vi "3Dconfig.vi"(0 "SceneObject in":refnum<vi>, 1 "Proximity Tap":bool, 2 "Weapon":T1(ring), 3 "error in (no error)":errorcluster) -> (5 "SceneObject out":refnum<vi>, 6 "error out":errorcluster)   [LabVIEW 2014]
doc: "Changes the appearance of the lightsaber. Specifically, this VI enables/disables the existing Lightsaber blade and changes the color"
uses:
  <vilib>/picture/3D Picture Control/NI_3D Picture Control.lvlib
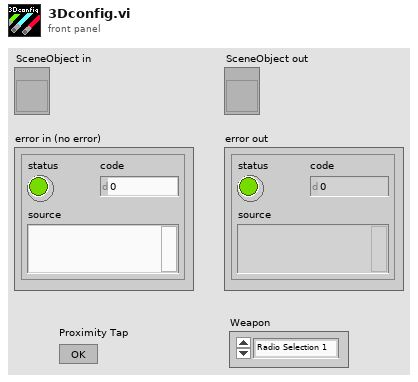
[diagram p1: front panel]
types:
  T1 = enum32{"Radio Selection 1", "Radio Selection 2", "Radio Selection 3", "Radio Selection 4"}
  T2 = enum16{"As a Decal", "With Modulation", "With Blending", "As a replacement"}
  T3 = typedef "imagedata.ctl" = cluster{"image type":i32, "image depth":i32, "image":u8[], "mask":u8[], "colors":u32[], "Rectangle":cluster{"left":i16, "top":i16, "right":i16, "bottom":i16}}
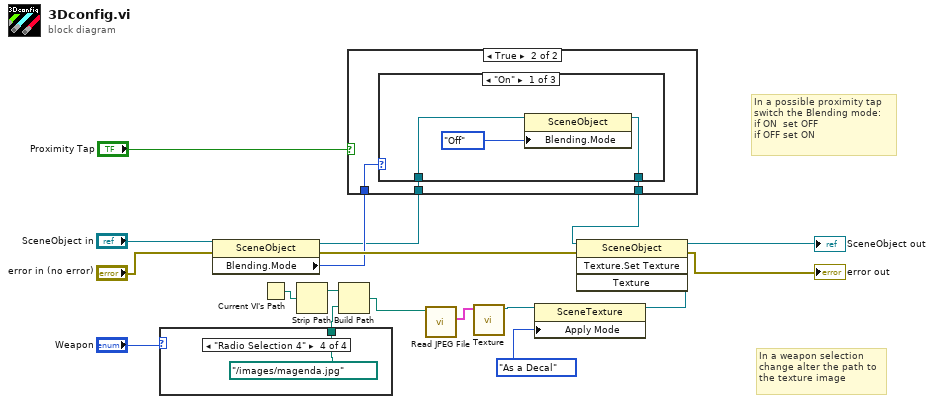
[diagram p0: block diagram]
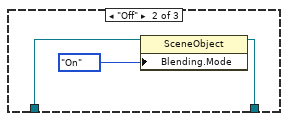
[diagram p3: hidden frame]
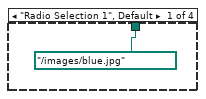
[diagram p5: hidden frame]
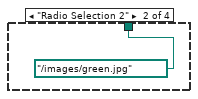
[diagram p6: hidden frame]
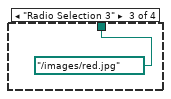
[diagram p7: hidden frame]
diagram:
  # "In a weapon selection\nchange alter the path to\nthe texture image"
  # "In a possible proximity tap\nswitch the Blending mode:\nif ON  set OFF\nif OFF set ON"
  n1 = case shown="\"Radio Selection 4\"" "Weapon" {
    tunnel: [path "../images/blue.jpg" ("path to JPEG file") path "../images/green.jpg" ("path to JPEG file") path "../images/red.jpg" ("path to JPEG file") path "../images/magenda.jpg" ("path to JPEG file")] -> w2
    frame "Radio Selection 1", Default {
    }
    frame "Radio Selection 2" {
    }
    frame "Radio Selection 3" {
    }
    frame "Radio Selection 4" {
    }
  }
  n2 = property on="Property Node" class="SceneObject"(reference="SceneObject in", error in="error in (no error)") -> (reference out=w6:refnum<vi>, error out=w12:errorcluster, "Blending.Mode"=w7:enum16{"Inherit Value", "Off", "On"})
  n3 = Current VI's Path() -> (path=w3:path)
  n4 = Strip Path(path=w3) -> (stripped path=w4:path)  [unwired: 1 out]
  n5 = Build Path(base path=w4, name or relative path=w2) -> (appended path=w1:path)
  n6 = case shown="True" "Proximity Tap" {
    tunnel: w7 -> [_ w26]
    tunnel: w6 -> [w23 w24]
    tunnel: [w23 w25] -> w5
    frame False {
    }
    frame True {
      n7 = case shown="\"On\"" w26 {
        tunnel: [w27 w31 w33] -> w25
        tunnel: w24 -> [w28 w30 w33]
        frame "On" {
          n8 = property on="Property Node" class="SceneObject"(reference=w28, "Blending.Mode"=enum16{"Inherit Value", "Off", "On"}."Off" ("Blending:Mode")) -> (reference out=w27:refnum<vi>)  [unwired: 1 in, 1 out]
        }
        frame "Off" {
          n9 = property on="Property Node" class="SceneObject"(reference=w30, "Blending.Mode"=enum16{"Inherit Value", "Off", "On"}."On" ("Blending:Mode")) -> (reference out=w31:refnum<vi>)  [unwired: 1 in, 1 out]
        }
        frame "Inherit Value" {
        }
      }
    }
  }
  n10 = call <vilib>:"Read JPEG File.vi"("path to JPEG file"=w1) -> ("image data"=w15:T3)  [unwired: 8 in, 2 out]
  n11 = call <vilib>:"Texture.vi"("Image"=w15) -> ("New Texture Refnum"=w17:refnum<vi>)  [unwired: 9 in, 1 out]
  n12 = property class="SceneTexture"(reference=w17, "Apply Mode"=T2."As a Decal") -> (reference out=w18:refnum<vi>)  [unwired: 1 in, 1 out]
  n13 = invoke class="SceneObject" method="Texture.Set Texture"(reference=w5, error in=w12, "Texture"=w18) -> (reference out=→"SceneObject out":refnum<vi>, error out=→"error out":errorcluster)  [unwired: 1 in, 2 out]
